vi "Thumbstick.vi"(7 "Analog Ref Override":dbl, 8 "Error In":errorcluster, 10 "Thumbstick Configuration":T1, 11 "LINX Resource":T3) -> (0 "Error Out":errorcluster, 2 "Thumbstick Data":T2, 3 "LINX Resource":T3)   [LabVIEW 2020, in "LMH-LINX.lvlib"]
doc: "Read the thumbstick position using two AI channels and thumbstick button using one DI channel."
uses:
  LMH-LINX.lvlib
  Private/Type Defs/LINX Ref.ctl
  Private/Type Defs/Platform.ctl
  Private/Type Defs/Interface.ctl
  Private/Device/Type Defs/LINX Device Config.ctl
  Private/Device/Type Defs/TCP Config.ctl
  Private/Device/Type Defs/Channels.ctl
  Private/Type Defs/Thumbstick Data.ctl
  Peripherals/Digital/Digital Read 1 Chan.vi
  Peripherals/Analog/Analog Read N Chans.vi
  Peripherals/Digital/Digital Read N Chans.vi
  Private/Local IO/LinxAnalogRead.vi
  Utilities/Check Channel.vi
  Private/Local IO/LinxDigitalRead.vi
  Private/Utilties/Generate Error.vi
  Private/Device/Device.lvlib
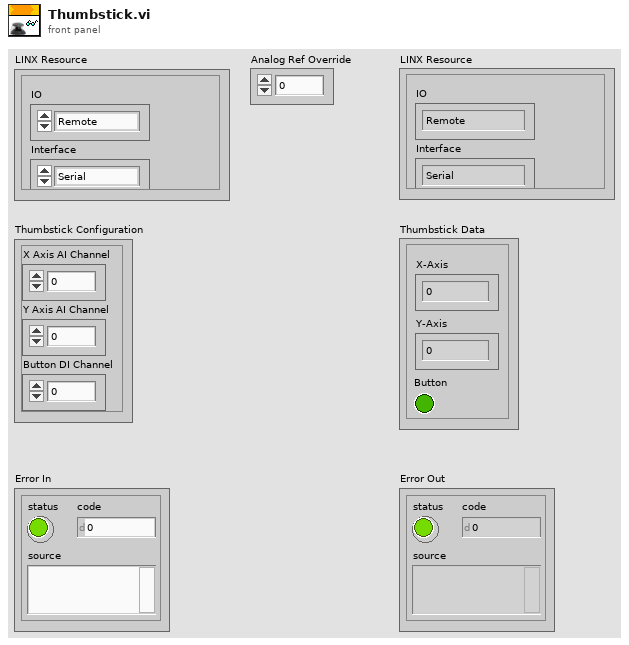
[diagram p1: front panel]
types:
  T1 = cluster{"X Axis AI Channel":u8, "Y Axis AI Channel":u8, "Button DI Channel":u8}
  T2 = typedef "LMH-LINX.lvlib/Thumbstick Data.ctl" = cluster{"X-Axis":dbl, "Y-Axis":dbl, "Button":bool}
  T3 = typedef "LMH-LINX.lvlib/LINX Ref.ctl" = cluster{"IO":T4, "Interface":T5, "LINX Device Config":T6}
  T4 = typedef "LMH-LINX.lvlib/Platform.ctl" = enum16{"Remote", "Local"}
  T5 = typedef "LMH-LINX.lvlib/Interface.ctl" = enum16{"Serial", "TCP"}
  T6 = typedef "LMH-LINX.lvlib/Device.lvlib/LINX Device Config.ctl" = cluster{"Interface":T5, "COM Port":refnum<visa-resource-name>, "TCP Configuration":T7, "Device Family":u8, "Device ID":u8, "Device Name":string, "TCP Ref":refnum<k5>, "Channels":T8}
  T7 = typedef "LMH-LINX.lvlib/Device.lvlib/TCP Config.ctl" = cluster{"IP Address":string, "Port":u16}
  T8 = typedef "LMH-LINX.lvlib/Channels.ctl" = cluster{"DI":u8[], "DO":u8[], "AI":u8[], "AO":u8[], "PWM":u8[], "QE":u8[], "UART":u8[], "I2C 2":u8[], "SPI":u8[], "CAN":u8[], "Servo":u8[], "AI Ref (V)":dbl, "AI Resolution (Bits)":u8, "AO Ref (V)":dbl, "AO Resolution (Bits)":u8}
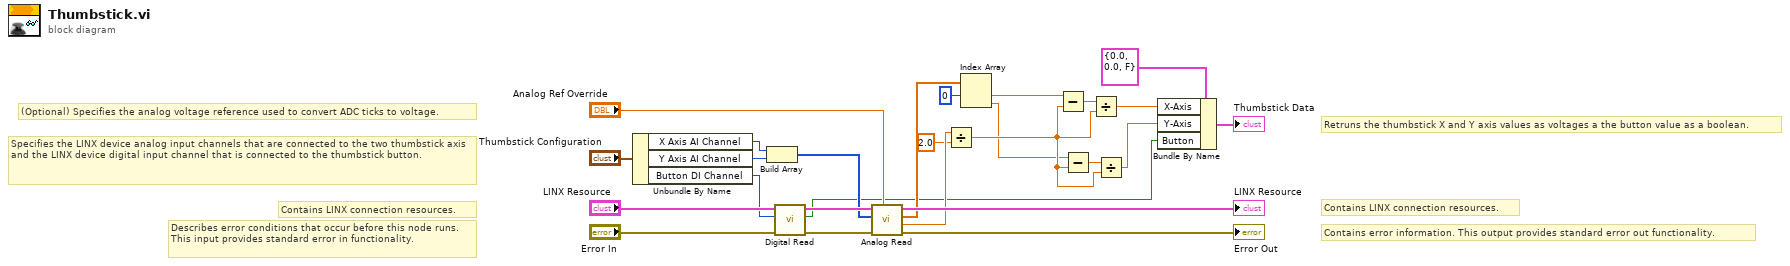
[diagram p0: block diagram]
diagram:
  # "Retruns the thumbstick X and Y axis values as voltages a the button value as a boolean."
  # "Specifies the LINX device analog input channels that are connected to the two thumbstick axis and the LINX device digital input channel that is connected to the thumbstick button."
  # "(Optional) Specifies the analog voltage reference used to convert ADC ticks to voltage."
  # "Contains LINX connection resources."
  # "Contains error information. This output provides standard error out functionality."
  # "Contains LINX connection resources."
  # "Describes error conditions that occur before this node runs. This input provides standard error in functionality."
  n1 = Unbundle By Name("Thumbstick Configuration") -> ("X Axis AI Channel"=w4:u8, "Y Axis AI Channel"=w3:u8, "Button DI Channel"=w2:u8)
  n2 = Build Array(w4, w3) -> (w24:u8[])
  n3 = call-poly "Digital Read.vi"("Error In"="Error In", "DI Channel"=w2, "LINX Resource"="LINX Resource") -> ("Error Out"=w25:errorcluster, "DI Value"=w1:bool, "LINX Resource"=w26:T3)  [unwired: 6 in]
  n4 = call-poly "Analog Read.vi"("Analog Ref Override"="Analog Ref Override", "Error In"=w25, "AI Channel(s)"=w24, "LINX Resource"=w26) -> ("Error Out"=→"Error Out":errorcluster, "AI Ref"=w16:dbl, "Voltages"=w17:dbl[], "LINX Resource"=→"LINX Resource":T3)  [unwired: 4 in]
  n5 = Divide(x=w16, y=2.0) -> (x/y=w12:dbl)
  n6 = Index Array(array=w17, index #1=0 ("index")) -> (element #1=w18:dbl, element #2=w11:dbl)  [unwired: 1 in]
  n7 = Subtract(x=w18, y=w12) -> (x-y=w14:dbl)
  n8 = Subtract(x=w11, y=w12) -> (x-y=w13:dbl)
  n9 = Divide(x=w14, y=w12) -> (x/y=w10:dbl)
  n10 = Divide(x=w13, y=w12) -> (x/y=w8:dbl)
  n11 = Bundle By Name(cluster=T2 {"X-Axis"=0.0, "Y-Axis"=0.0, "Button"=FALSE} ("Thumbstick Data"), "X-Axis"=w10, "Y-Axis"=w8, "Button"=w1) -> (→"Thumbstick Data":T2)
